vi "ReadyToKick.vi"(0 "object in":refnum<class "PassTactic.lvclass">, 5 "error in (no error)":errorcluster) -> (14 "object out":refnum<class "PassTactic.lvclass">, 16 "ready":bool, 19 "error out":errorcluster)   [LabVIEW 2023, in "PassTactic.lvclass"]
uses:
  PassTactic.lvclass
  Robot_class/tactics.ctl
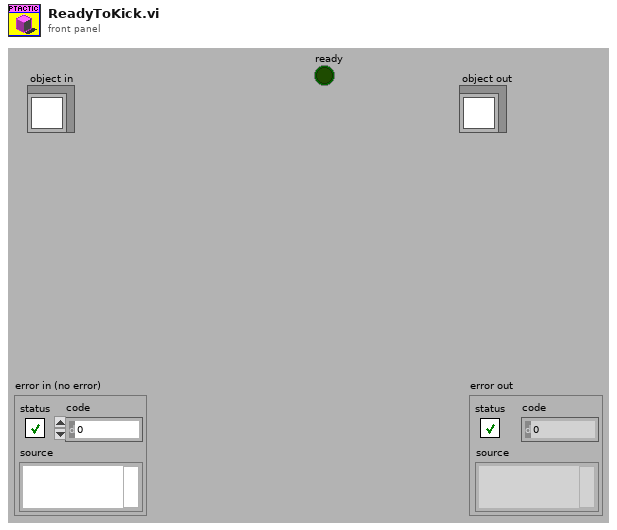
[diagram p1: front panel]
types:
  T1 = typedef "tactics.ctl" = enum16{"GoToBallPlacementPosition", "PlaceBall", "GoToBallPlacement", "5Robots", "BallPlacementEnemy", "ReceivePassInFuturePoint", "Roller", "PrepareRollToPassRollerGoTo", "PrepareRollToPassReceiverGoTo", "WaitRoll", "PositionToRoll", "PenaltyAttacker", "PassObserver", "PenaltyDefense", "TableReceiverTactic", "Test", "DefendGoal", "Marker", "FollowAttacker", "DefendArea", "Shoot", "AttackerAimGoal", "AttackerBallOutOfField", "AttackerBlock", "AttackerStop", "Duelist", "Halt", "ZigZag", "GoTo", "Timeout", "KickToBestRobot", "KickToPassReceiver", "PositionToReceivePass", "WaitPass", "Position", "Intercept", "PrepareShot", "Pass"}
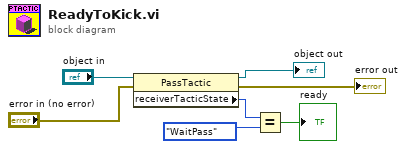
[diagram p0: block diagram]
diagram:
  n1 = property class="PassTactic"(reference="object in", error in="error in (no error)") -> (reference out=→"object out":refnum<class "PassTactic.lvclass">, error out=→"error out":errorcluster, "receiverTacticState "=w6:T1)
  n2 = Equal?(x=w6, y=tactics."WaitPass") -> (x = y?=→"ready":bool)
